vi "AT Initialise Library A.vi"(8 "error in (no error)":errorcluster) -> (0 "error out":errorcluster, 3 "Status":i32)   [LabVIEW 2019]
doc: "InitialiseLibrary\n\nOutput:\n I32 Status\n\nInput:\n void\n\nThis allows the SDK to setup its internal data structures and to detect any cameras that are attached."
uses:
  atcoreA.dll
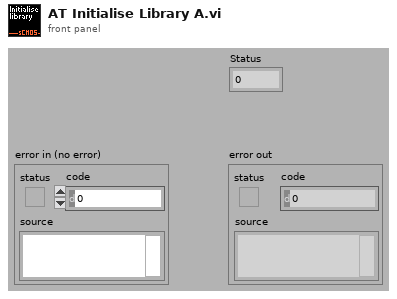
[diagram p1: front panel]
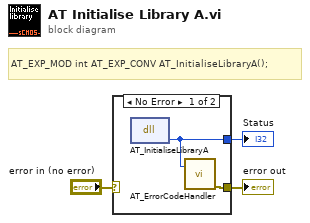
[diagram p0: block diagram]
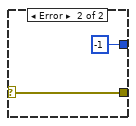
[diagram p2: hidden frame]
diagram:
  # "AT_EXP_MOD int AT_EXP_CONV AT_InitialiseLibraryA();"
  n1 = case shown="No Error" "error in (no error)" {
    selector: "error in (no error)" -> [_ w7]
    tunnel: [w4 -1] -> w1
    tunnel: [w5 w7] -> w2
    frame No Error {
      n2 = dll-call lib="atcoreA.dll" fn="AT_InitialiseLibraryA"() -> ("Status"=w4:i32)  [unwired: 3 in, 2 out]
      n3 = call "AT_ErrorCodeHandler.vi"("Error"=w4) -> ("error out"=w5:errorcluster)  [unwired: 6 in]
    }
    frame Error {
    }
  }
  "Status" <- w1
  "error out" <- w2
